vi "Update Stats.vi"(8 "error in (no error)":errorcluster, 10 "Team Stats":T1[](array[typedef]), 11 "Dashboard Panel in":refnum<class "Dashboard Panel.lvclass">) -> (0 "error out":errorcluster, 3 "Dashboard Panel out":refnum<class "Dashboard Panel.lvclass">)   [LabVIEW 2020, in "SB App.lvlib" / "Dashboard Panel.lvclass"]
uses:
  Dashboard Panel.lvclass
  Team Status Data.ctl
  SquareBattle/Team Stats.ctl
  SquareBattle/Team State.ctl
  Dashboard Panel.lvclass/Dashboard Panel.ctl
  SB App.lvlib
  SquareBattle/SquareBattle.lvlib
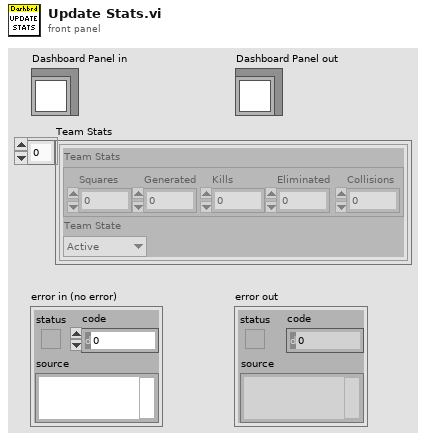
[diagram p1: front panel]
types:
  T1 = typedef "SB App.lvlib/Team Status Data.ctl" = cluster{"Team Stats":T2, "Team State":T3}
  T2 = typedef "SquareBattle.lvlib/Team Stats.ctl" = cluster{"Squares":i32, "Generated":i32, "Kills":i32, "Eliminated":i32, "Collisions":i32}
  T3 = typedef "SquareBattle.lvlib/Team State.ctl" = enum16{"Active", "Defeated", "Won"}
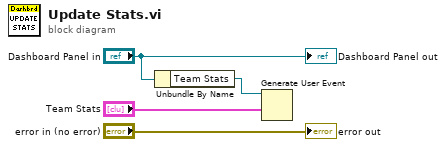
[diagram p0: block diagram]
diagram:
  n1 = Unbundle By Name("Dashboard Panel in") -> ("Team Stats"=w2:refnum<user-event>)
  n2 = Generate User Event(user event=w2, event data cluster="Team Stats") -> ()  [unwired: 2 in, 2 out]
  "error out" <- "error in (no error)"
  "Dashboard Panel out" <- "Dashboard Panel in"
